vi "GetOneDigitalValue.vi"(8 "error in (no error)":errorcluster, 10 "wValue":i16, 11 "wIndex":i16) -> (0 "error out":errorcluster, 2 "wValue out":i16, 3 "function return":i16)   [LabVIEW 2013, in "HS3AcquireData.lvlib"]
doc: "Description: This routine transfers a single digital input value from the memory in the DLL to the memory of the application.\n\nInput: wIndex The index of the measured data point, relative\nto the trigger point (negative for pre samples, positive for post samples)\nOutput: wValue Return address for the digital input value.\nReturn value E_NO_ERRORS | E_NOT_SUPPORTED | E_NO_HARDWARE\n\nFunction prototype: word GetOneDigitalValue( word wIndex, word *wValue )\n\nshort int GetOneDigitalValue ( short int wIndex, short int *wValue );"
uses:
  HS3AcquireData.lvlib
  hs3.dll
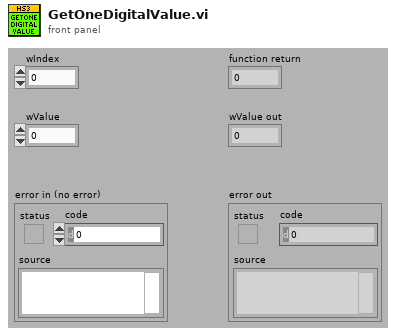
[diagram p1: front panel]
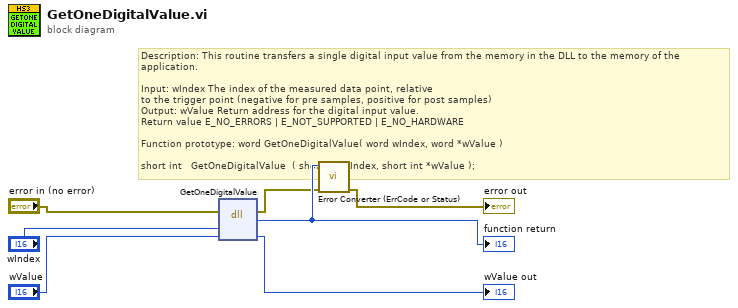
[diagram p0: block diagram]
diagram:
  # "Description: This routine transfers a single digital input value from the memory in the DLL to the memory of the application.\n\nInput: wIndex The index of the measured data point, relative\nto the trigger point (negative for pre samples, positive for post samples)\nOutput: wValue Return address for the digital input value.\nReturn value E_NO_ERRORS | E_NOT_SUPPORTED | E_NO_HARDWARE\n\nFunction prototype: word GetOneDigitalValue( word wIndex, word *wValue )\n\nshort int \t\tGetOneDigitalValue\t\t( short int wIndex, short int *wValue );"
  n1 = dll-call lib="C:/Documents and Settings/admin/Pulpit/HS3 LabViewLib/HS3_WRAPPER/AcquireData/hs3.*" fn="GetOneDigitalValue"(error in="error in (no error)", "wIndex"="wIndex", "wValue"="wValue") -> (error out=w2:errorcluster, w7:i16, "wValue"=→"wValue out":i16)  [unwired: 3 in, 1 out]
  "function return" <- w7
  n2 = call "Error Converter (ErrCode or Status).vi"("error in (no error)"=w2, "error code"=w7) -> ("error out"=→"error out":errorcluster)  [unwired: 9 in]
